vi "SQLite Query - Delete.vi"(6 "A[Strings] Value":string[](array[string]), 7 "A[Strings]":string[](array[string]), 8 "error in":errorcluster, 10 "Table Headers":string[](array[string]), 11 "Table Name":string) -> (0 "error out":errorcluster, 3 "SQLite Query":string)   [LabVIEW 2014, in "TableLogger_SQLite_Actor.lvlib" / "TableLogger_SQLite_Actor.lvclass"]
uses:
  TableLogger_SQLite_Actor.lvclass
  TableLogger_CSV_Actor/TableLogger_CSV_Actor/TableLogger_CSV_Actor.lvclass
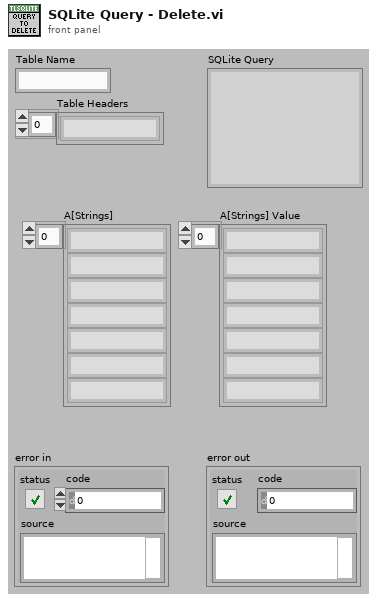
[diagram p1: front panel]
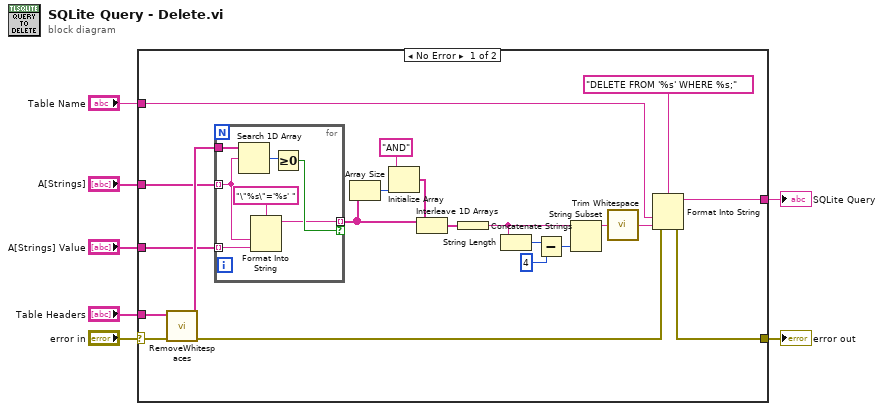
[diagram p0: block diagram]
diagram:
  n1 = case shown="No Error" "error in" {
    selector: "error in" -> [w27 w36]
    tunnel: "Table Name" -> [w13 _]
    tunnel: "Table Headers" -> [w28 _]
    tunnel: [w8 w36] -> w4
    tunnel: [w12 _] -> w3
    tunnel: "A[Strings]" -> [w11 _]
    tunnel: "A[Strings] Value" -> [w10 _]
    frame No Error {
      n2 = call "RemoveWhitespaces.vi"("error in (no error)"=w27, "Array In"=w28) -> ("error out"=w9:errorcluster, "Array removing empty space"=w14:string[])  [unwired: 8 in]
      n3 = for {
        tunnel: w14 -> [w35]
        tunnel: w11 -> [w30] mode=indexing
        tunnel: w10 -> [w31] mode=indexing
        tunnel: [w29] -> w17 mode=indexing if=w33
        n4 = Search 1D Array(1D array=w35, element=w30) -> (index of element=w34:i32)  [unwired: 1 in]
        n5 = Format Into String(format string="\"%s\"='%s' ", w30, w31) -> (resulting string=w29:string)  [unwired: 2 in, 1 out]
        n6 = Greater Or Equal To 0?(x=w34) -> (x >= 0?=w33:bool)
      }
      n7 = Array Size(array=w17) -> (size(s)=w21:i32)
      n8 = Initialize Array("AND" ("format string"), w21) -> (w19:string[])
      n9 = Interleave 1D Arrays(w17, w19) -> (w20:string[])
      n10 = Concatenate Strings(w20) -> (w23:string)
      n11 = String Length(string=w23) -> (length=w24:i32)
      n12 = Subtract(x=w24, y=4) -> (x-y=w25:i32)
      n13 = String Subset(string=w23, length (rest)=w25) -> (substring=w22:string)  [unwired: 1 in]
      n14 = call <vilib>:"Trim Whitespace.vi"("string"=w22) -> ("trimmed string"=w16:string)  [unwired: 1 in]
      n15 = Format Into String(format string="DELETE FROM '%s' WHERE %s;" ("SQL"), error in=w9, w13, w16) -> (resulting string=w12:string, error out=w8:errorcluster)  [unwired: 1 in]
    }
    frame Error {
    }
  }
  "SQLite Query" <- w3
  "error out" <- w4
